vi "Eagle Find Spot Pixel.vi"(7 "Load From File":bool, 8 "error in":errorcluster, 10 "Picture Path":path=path "C:/DC Results", 11 "Image":T1(plugin-control)) -> (0 "error out":errorcluster, 2 "Y Pixel":i32, 3 "X Pixel":i32)   [LabVIEW 2015]
panel:
  out "Max Index":i32
  out "Max Value":u16
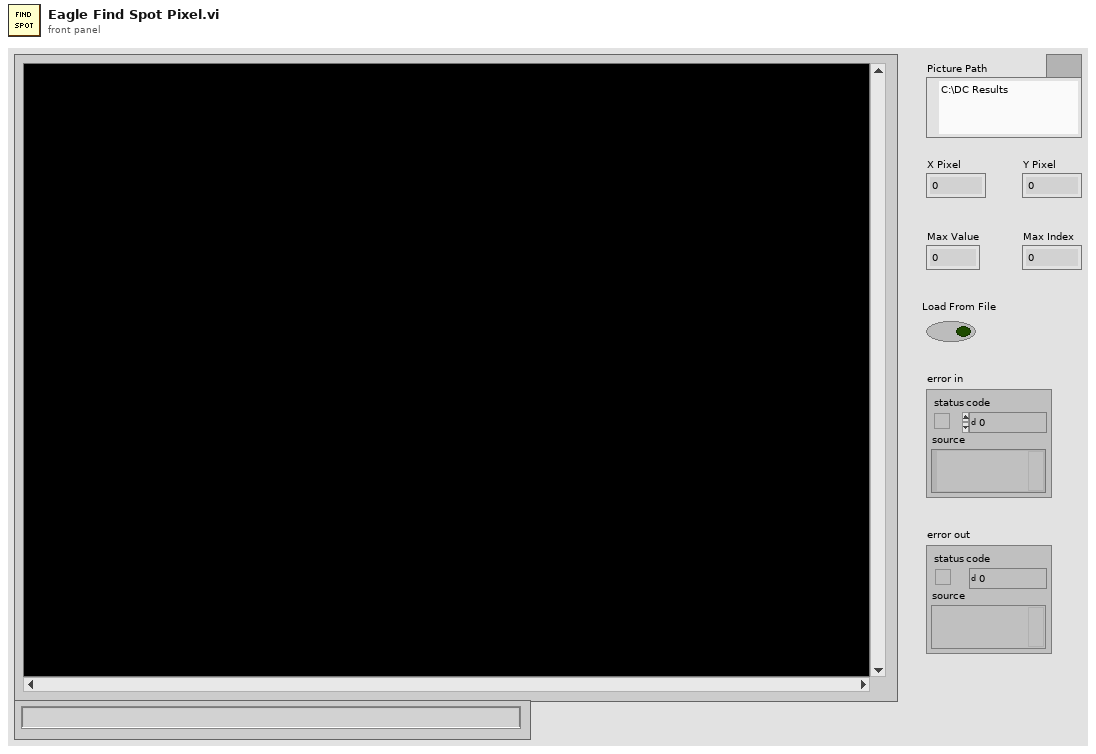
[diagram p1: front panel]
types:
  T1 = typedef "IMAQ Image.ctl" = refnum<image>
  T2 = typedef "Image Type" = u32
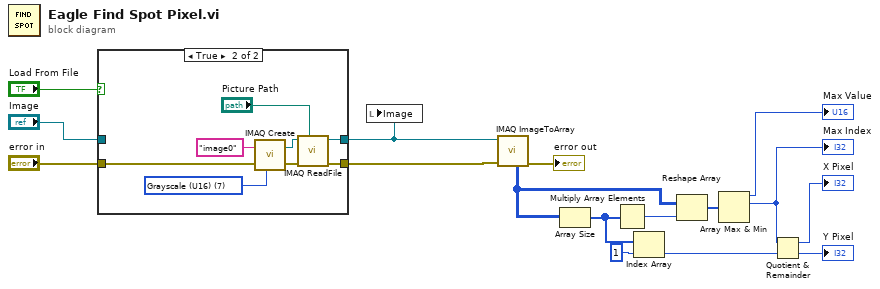
[diagram p0: block diagram]
diagram:
  n1 = case shown="True" "Load From File" {
    tunnel: [w18 w21] -> w2
    tunnel: "Image" -> [w18 _]
    tunnel: [w17 w23] -> w1
    tunnel: "error in" -> [w17 w22]
    frame False {
    }
    frame True {
      w19 = T2 7 items=["Grayscale (U8)", "Grayscale (I16)", "Grayscale (SGL)", "Complex (CSG)", "RGB (U32)", "HSL (U32)", "RGB (U64)", "Grayscale (U16)"] ("Image Type")
      n2 = call "IMAQ Create"("Image Name"="image0", "Image Type"=w19, "error in (no error)"=w22) -> ("New Image"=w25:T1, "error out"=w26:errorcluster)  [unwired: 2 in]
      n3 = call "IMAQ ReadFile"("File Path"="Picture Path", "error in (no error)"=w26, "Image"=w25) -> ("error out"=w23:errorcluster, "Image Out"=w21:T1)  [unwired: 4 in, 3 out]
    }
  }
  n4 = local write "Image"(w2) -> ()
  n5 = call "IMAQ ImageToArray"("error in (no error)"=w1, "Image"=w2) -> ("Image Pixels (U16)"=w3:u16[][], "error out"=→"error out":errorcluster)  [unwired: 2 in, 3 out]
  n6 = Array Size(array=w3) -> (size(s)=w12:i32[])
  n7 = Multiply Array Elements(1:w12) -> (0:w16:i32)
  n8 = Index Array(array=w12, index=1) -> (element=w10:i32)
  n9 = Reshape Array(w3, w16) -> (w15:u16[])
  n10 = Array Max & Min(array=w15) -> (max value=→"Max Value":u16, max index (indices)=w13:i32)  [unwired: 2 out]
  "Max Index" <- w13
  n11 = Quotient & Remainder(x=w13, y=w10) -> (x-y*floor(x/y)=→"X Pixel":i32, floor(x/y)=→"Y Pixel":i32)
